vi "Test Simon Engine.vi"() -> ()   [LabVIEW 2019]
uses:
  Simon_Engine.lvclass
panel:
  out "Level":i32
  out "Yellow":bool
  out "Green":bool
  out "Red":bool
  out "Blue":bool
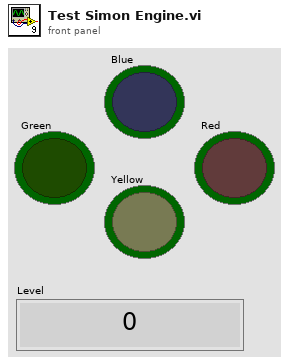
[diagram p1: front panel]
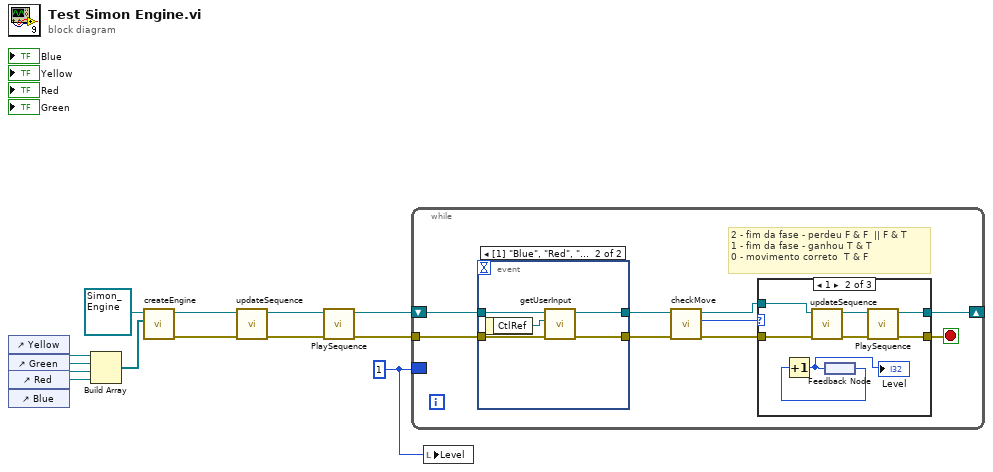
[diagram p0: block diagram]
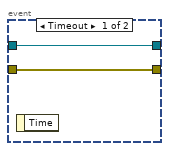
[diagram p2: hidden frame]
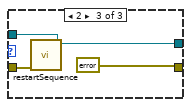
[diagram p4: hidden frame]
diagram:
  w1 = 1
  n1 = control-ref of="Yellow"() -> (w9:refnum<vi>)
  n2 = control-ref of="Green"() -> (w8:refnum<vi>)
  n3 = control-ref of="Red"() -> (w7:refnum<vi>)
  n4 = control-ref of="Blue"() -> (w6:refnum<vi>)
  n5 = Build Array(w9, w8, w7, w6) -> (w5:refnum<vi>[])
  n6 = call-dynamic "createEngine.vi"("ledRefnums"=w5, "Simon_Engine in"=refnum<class "Simon_Engine.lvclass"> refnum) -> ("error out"=w12:errorcluster, "Simon_Engine out"=w11:refnum<class "Simon_Engine.lvclass">)  [unwired: 8 in]
  n7 = call-dynamic "updateSequence.vi"("error in (no error)"=w12, "Simon_Engine in"=w11) -> ("error out"=w10:errorcluster, "Simon_Engine out"=w3:refnum<class "Simon_Engine.lvclass">)  [unwired: 8 in]
  n8 = call-dynamic "PlaySequence.vi"("error in (no error)"=w10, "Simon_Engine in"=w3) -> ("error out"=w4:errorcluster, "Simon_Engine out"=w2:refnum<class "Simon_Engine.lvclass">)  [unwired: 8 in]
  n9 = while {
    tunnel: w4 -> [w22]
    shift-right: [w17] -> _
    shift-left: w2 -> [w15]
    border: w1 -> [_]
    stop <- w20 stop-if-true
    # "2 - fim da fase - perdeu F & F  || F & T\n1 - fim da fase - ganhou T & T\n0 - movimento correto  T & F"
    n10 = event shown="[1] \"Blue\", \"Red\", \"Green\", \"Yellow\": Mouse Down" {
      selector: _ -> [_ _]
      dyn-events: _ -> [_ _]
      timeout: _ -> [_ _]
      tunnel: w22 -> [w24 w29]
      tunnel: [w24 w28] -> w16
      tunnel: w15 -> [w23 w27]
      tunnel: [w23 w26] -> w14
      event Timeout {
        n11 = event-data() -> ()  [unwired: 1 in, 1 out]
      }
      event "Blue", "Red", "Green", "Yellow": Mouse Down {
        n12 = event-data() -> ("CtlRef"=w25:refnum<vi>)  [unwired: 1 in]
        n13 = call-dynamic "getUserInput.vi"("error in (no error)"=w29, "clickedLEDReference"=w25, "Simon_Engine in"=w27) -> ("error out"=w28:errorcluster, "Simon_Engine out"=w26:refnum<class "Simon_Engine.lvclass">)  [unwired: 7 in]
      }
    }
    n14 = call-dynamic "checkMove.vi"("error in (no error)"=w16, "Simon_Engine in"=w14) -> ("error out"=w21:errorcluster, "MachStatus"=w18:i16, "Simon_Engine out"=w19:refnum<class "Simon_Engine.lvclass">)  [unwired: 7 in]
    n15 = case shown="1" w18 {
      tunnel: w21 -> [w30 w39 w43]
      tunnel: [w30 w36 errorcluster {"status"=TRUE, "code"=0, "source"=""} ("error out")] -> w20
      tunnel: w19 -> [w31 w37 w42]
      tunnel: [w31 w34 w41] -> w17
      frame 0, Default {
      }
      frame 1 {
        n16 = call-dynamic "updateSequence.vi"("error in (no error)"=w39, "Simon_Engine in"=w37) -> ("error out"=w38:errorcluster, "Simon_Engine out"=w35:refnum<class "Simon_Engine.lvclass">)  [unwired: 8 in]
        n17 = feedback #1() -> (w33:i32)
        n18 = Increment(x=w33) -> (x+1=w32:i32)
        "Level" <- w32
        n19 = feedback-in #1(w32) -> ()
        n20 = call-dynamic "PlaySequence.vi"("error in (no error)"=w38, "Simon_Engine in"=w35) -> ("error out"=w36:errorcluster, "Simon_Engine out"=w34:refnum<class "Simon_Engine.lvclass">)  [unwired: 8 in]
      }
      frame 2 {
        n21 = call-dynamic "restartSequence.vi"("error in (no error)"=w43, "Simon_Engine in"=w42) -> ("Simon_Engine out"=w41:refnum<class "Simon_Engine.lvclass">)  [unwired: 8 in, 1 out]
      }
    }
  }
  n22 = local write "Level"(w1) -> ()
